vi "DutInit.vi"(5 "Active Dut":T1, 7 "Response Timeout (ms)":i32 min=0, 8 "Error In":errorcluster, 9 "Initial PAC (Hex)":string, 10 "Device ID (Hex)":string, 11 "FPGA VI Reference In":refnum<k20>) -> (0 "Error Out":errorcluster, 1 "ID|PAC OK":bool, 2 "Initial PAC Out":string, 3 "Elements Remaining":u32, 4 "Credentials":string, 6 "Init Resp":string)   [LabVIEW 2018]
uses:
  Resources_Test/UART/ControlTestSlot.ctl
panel:
  out "Device ID Out":string
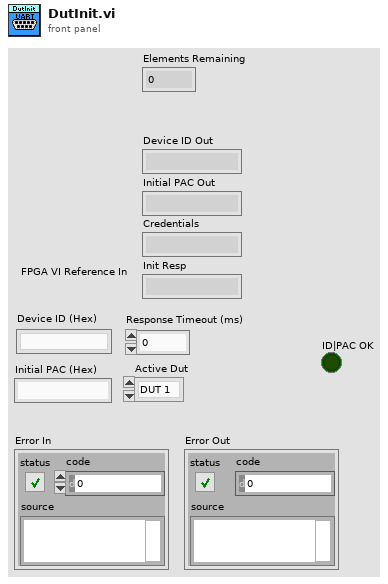
[diagram p1: front panel]
types:
  T1 = typedef "ControlTestSlot.ctl" = enum16{"DUT 1", "DUT 2"}
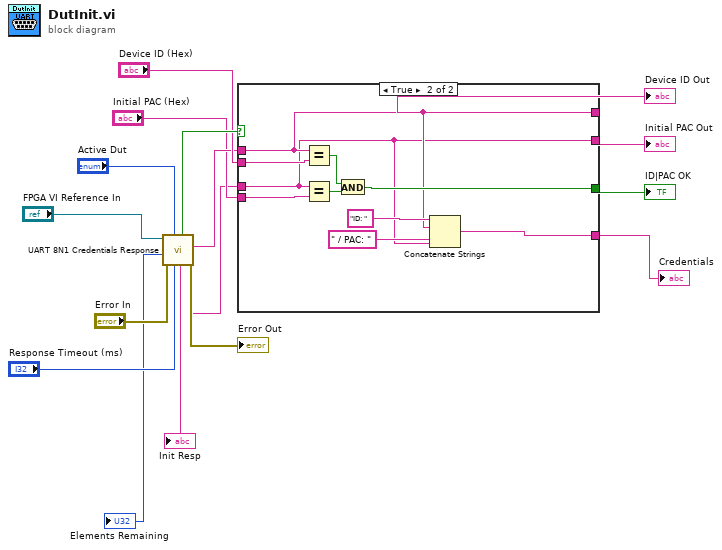
[diagram p0: block diagram]
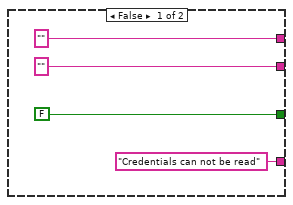
[diagram p2: hidden frame]
diagram:
  n1 = call "UART 8N1 Credentials Response.vi"("Response Timeout (ms)"="Response Timeout (ms)", "Enum"="Active Dut", "Error In"="Error In", "FPGA VI Reference In"="FPGA VI Reference In") -> ("Error Out"=→"Error Out":errorcluster, "Initial PAC (Hex)"=w9:string, "Device ID (Hex)"=w11:string, "Init Resp"=→"Init Resp":string, "Get Cred OK"=w13:bool, "Elements Remaining"=→"Elements Remaining":u32)  [unwired: 1 in, 1 out]
  n2 = case shown="True" w13 {
    tunnel: "Device ID (Hex)" -> [_ w30]
    tunnel: w11 -> [_ w24]
    tunnel: "Initial PAC (Hex)" -> [_ w29]
    tunnel: w9 -> [_ w21]
    tunnel: [FALSE w28] -> w7
    tunnel: ["" ("Device ID (Hex)") w24] -> w6
    tunnel: ["" ("Initial PAC (Hex)") w21] -> w5
    tunnel: ["Credentials can not be read" w22] -> w4
    frame False {
    }
    frame True {
      n3 = Equal?(x=w24, y=w30) -> (x = y?=w27:bool)
      n4 = Equal?(x=w21, y=w29) -> (x = y?=w26:bool)
      n5 = And(x=w27, y=w26) -> (x .and. y?=w28:bool)
      n6 = Concatenate Strings("ID: " ("string"), w24, " / PAC: " ("string"), w21) -> (w22:string)
    }
  }
  "ID|PAC OK" <- w7
  "Device ID Out" <- w6
  "Initial PAC Out" <- w5
  "Credentials" <- w4
